vi "读取Info.vi"(8 "error in (no error)":errorcluster caption="错误输入（无错误）", 11 "单例输入":refnum<class "单例.lvclass">) -> (0 "error out":errorcluster caption="错误输出", 2 "Info":string, 3 "单例输出":refnum<class "单例.lvclass">)   [LabVIEW 2011, in "单例.lvlib" / "单例.lvclass"]
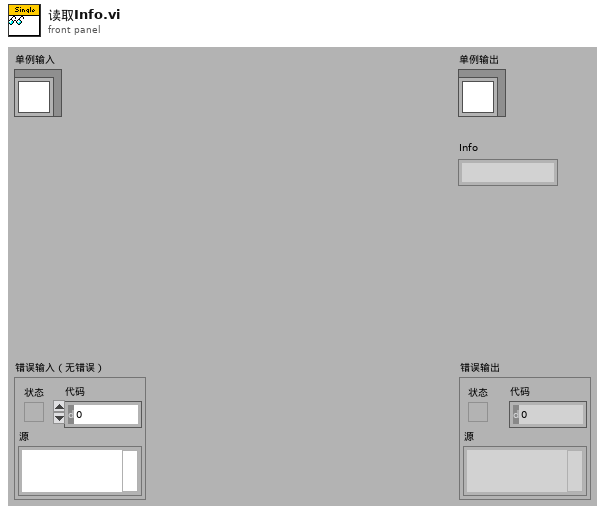
[diagram p1: front panel]
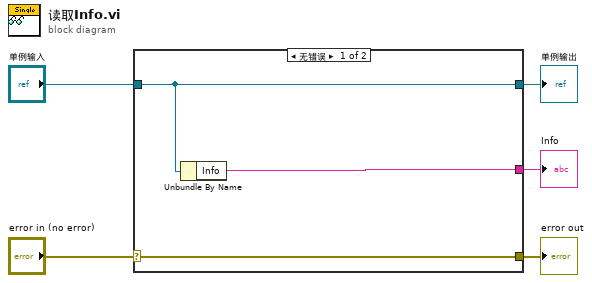
[diagram p0: block diagram]
diagram:
  n1 = case shown="无错误" "error in (no error)" {
    selector: "error in (no error)" -> [w8 w9]
    tunnel: [w8 w9] -> w4
    tunnel: [w7 w10] -> w2
    tunnel: "单例输入" -> [w7 w10]
    tunnel: [w6 _] -> w1
    frame No Error {
      n2 = Unbundle By Name(w7) -> ("Info"=w6:string)
    }
    frame Error {
    }
  }
  "error out" <- w4
  "单例输出" <- w2
  "Info" <- w1
